vi "Populate Example Description.vi"(5 "API Dir":path[](array[path]), 6 "Cluster":cluster{"Force?(F)":bool, "Show FP":bool}={"Force?(F)"=FALSE, "Show FP"=TRUE}, 7 "doc dir":path[](array[path]), 8 "error in (no error)":errorcluster, 10 "Language Ring":string(combo)="English(en-us)") -> (0 "error out":errorcluster)   [LabVIEW 2017, in "csmdoc.lvlib"]
uses:
  csmdoc.lvlib
  BEditor-PopoulateExampleDesc.vi
  _Typedef/DocElement.ctl
  _Shared/CSM Shared.lvlib
  Communicable State Machine.lvlib
  _tool/_batchEditorDialog/batchEditorDialog.lvlib
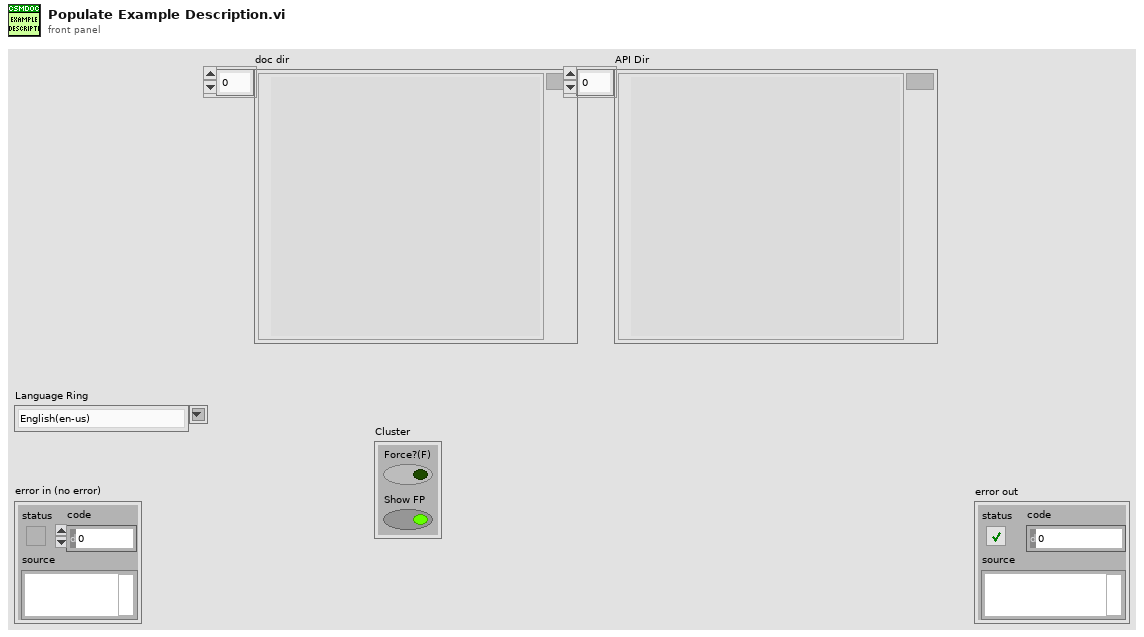
[diagram p1: front panel]
types:
  T1 = typedef "csmdoc.lvlib/DocNote.ctl" = cluster{"ID":string, "Content":string, "Type":string}
  T2 = typedef "csmdoc.lvlib/DocElement.ctl" = cluster{"ID":string, "Content":string[], "SubIDs":string[], "Path":string[]}
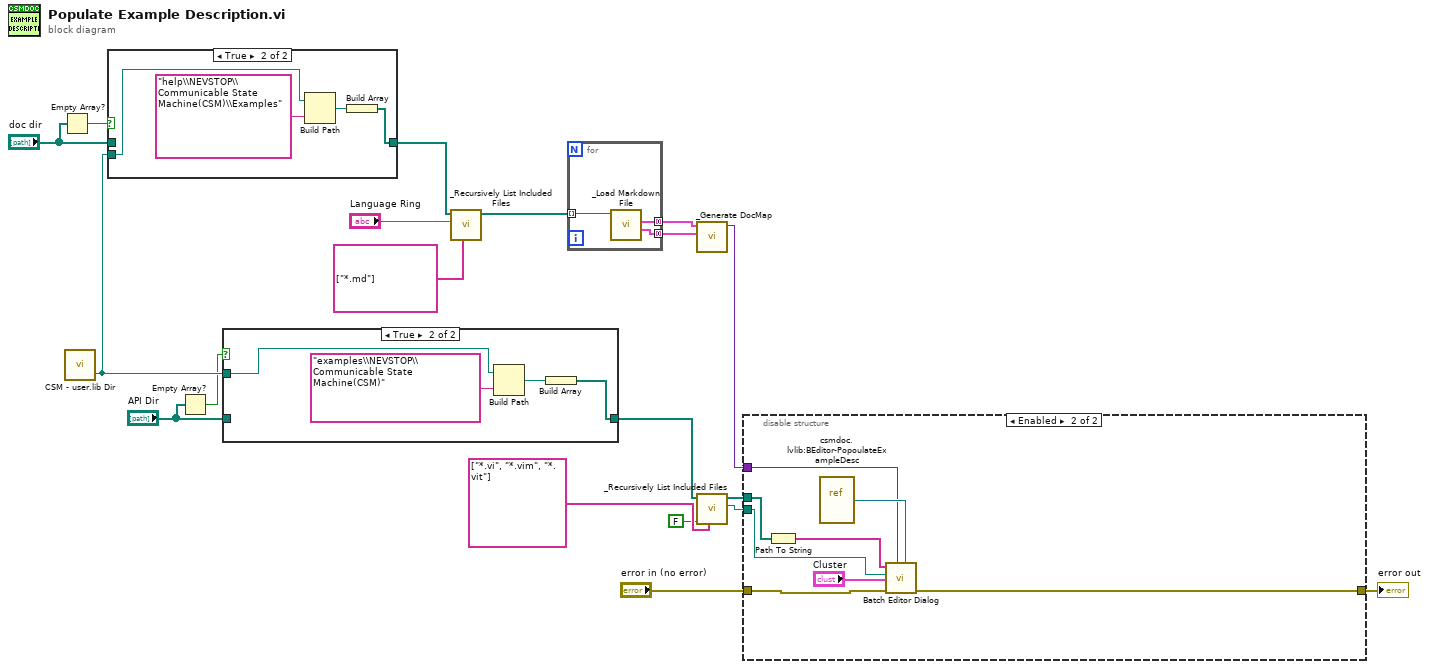
[diagram p0: block diagram]
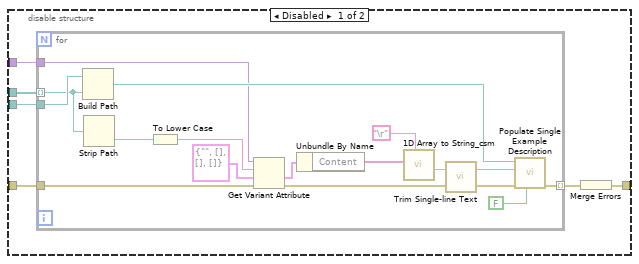
[diagram p2: hidden frame]
diagram:
  n1 = Empty Array?(array="doc dir") -> (empty?=w14:bool)
  n2 = call "CSM - user.lib Dir.vi"() -> ("<LabVIEW>"=w16:path)  [unwired: 2 in, 1 out]
  n3 = case shown="True" w14 {
    tunnel: [w20 w21] -> w9
    tunnel: w16 -> [_ w22]
    tunnel: "doc dir" -> [w20 _]
    frame False {
    }
    frame True {
      n4 = Build Path(base path=w22, name or relative path="help\\NEVSTOP\\Communicable State Machine(CSM)\\Examples") -> (appended path=w23:path)
      n5 = Build Array(w23) -> (w21:path[])
    }
  }
  n6 = Empty Array?(array="API Dir") -> (empty?=w12:bool)
  n7 = case shown="True" w12 {
    tunnel: [w25 w26] -> w3
    tunnel: w16 -> [_ w27]
    tunnel: "API Dir" -> [w25 _]
    frame False {
    }
    frame True {
      n8 = Build Path(base path=w27, name or relative path="examples\\NEVSTOP\\Communicable State Machine(CSM)") -> (appended path=w28:path)
      n9 = Build Array(w28) -> (w26:path[])
    }
  }
  n10 = call "_Recursively List Included Files.vi"("pattern"=string[] ["*.md"], "Language Ring"="Language Ring", "dir"=w9) -> ("Array"=w6:path[])  [unwired: 7 in, 1 out]
  n11 = for {
    tunnel: w6 -> [w32] mode=indexing
    tunnel: [w31] -> w19 mode=concatenating
    tunnel: [w30] -> w18 mode=concatenating
    n12 = call "_Load Markdown File.vi"("Path"=w32) -> ("Array 2"=w30:T1[], "Array"=w31:T2[])  [unwired: 8 in, 1 out]
  }
  n13 = call "_Generate DocMap.vi"("Array 2"=w18, "Array"=w19) -> ("Variant"=w17:variant)  [unwired: 9 in]
  n14 = call "_Recursively List Included Files.vi"("pattern"=string[] ["*.vi", "*.vim", "*.vit"], "apply _ filter?(T)"=FALSE, "dir"=w3) -> ("Common Path"=w2:path, "Array"=w1:path[])  [unwired: 7 in]
  n15 = disable-structure shown="Enabled" {
    disable-tunnel: w2 -> [w38 w56]
    disable-tunnel: w17 -> [w37 w57]
    disable-tunnel: w1 -> [w36 w55]
    disable-tunnel: "error in (no error)" -> [w35 w58]
    disable-tunnel: [w33 w59] -> w15
    frame Disabled {
      n16 = for {
        tunnel: w38 -> [w44]
        tunnel: w37 -> [w43]
        tunnel: w36 -> [w42] mode=indexing
        tunnel: [w41] -> w34 mode=indexing
        tunnel: w35 -> [w39]
        n17 = Build Path(base path=w44, name or relative path=w42) -> (appended path=w48:path)
        n18 = Strip Path(path=w42) -> (name=w54:string)  [unwired: 1 out]
        n19 = To Lower Case(string=w54) -> (all lower case string=w53:string)
        n20 = Get Variant Attribute(Variant=w43, name=w53, default value (empty Variant)=T2 {"ID"="", "Content"=[], "SubIDs"=[], "Path"=[]} ("Cluster"), error in=w39) -> (value=w51:T2, error out=w40:errorcluster)  [unwired: 2 out]
        n21 = Unbundle By Name(w51) -> ("Content"=w50:string[])
        n22 = call "1D Array to String_csm.vi"("delimiter (Tab)"="\r", "Array of Strings"=w50) -> ("delimited string"=w46:string)  [unwired: 9 in]
        n23 = call "Trim Single-line Text.vi"("single-line text"=w46) -> ("trimed text"=w45:string)  [unwired: 2 in]
        n24 = call "Populate Single Example Description.vi"("Show FP"=FALSE, "error in (no error)"=w40, "VI Description"=w45, "Path"=w48) -> ("error out"=w41:errorcluster)  [unwired: 7 in]
      }
      n25 = Merge Errors(w34) -> (w33:errorcluster)
    }
    frame Enabled {
      n26 = Path To String(path=w55) -> (string=w62:string[])
      n27 = vi-ref "csmdoc.lvlib:BEditor-PopoulateExampleDesc.vi"() -> (w61:refnum<vi>)
      n28 = call "Batch Editor Dialog.vi"("VI Refnum"=w61, "Reference"=w57, "Error in"=w58, "Option"="Cluster", "Root"=w56, "Entries"=w62) -> ("Error out"=w59:errorcluster)  [unwired: 5 in]
    }
  }
  "error out" <- w15
